vi "Launch Worker.vi"(8 "error in (no error)":errorcluster, 9 "Name":string, 10 "Subordinate Object":refnum<class "Worker.lvclass">, 11 "Application Controller in":refnum<class "Application Controller.lvclass">) -> (0 "error out":errorcluster, 2 "Nested Actor's Enqueuer":refnum<class "Message Enqueuer.lvclass">, 3 "Application Controller out":refnum<class "Application Controller.lvclass">)   [LabVIEW 2016, in "Application Controller.lvclass"]
uses:
  Application Controller.lvclass
  Worker/Worker.lvclass
  C:/github/Measure_core/Template Module/Template Module.lvclass
  <vilib>/ActorFramework/Message Enqueuer/Message Enqueuer.lvclass
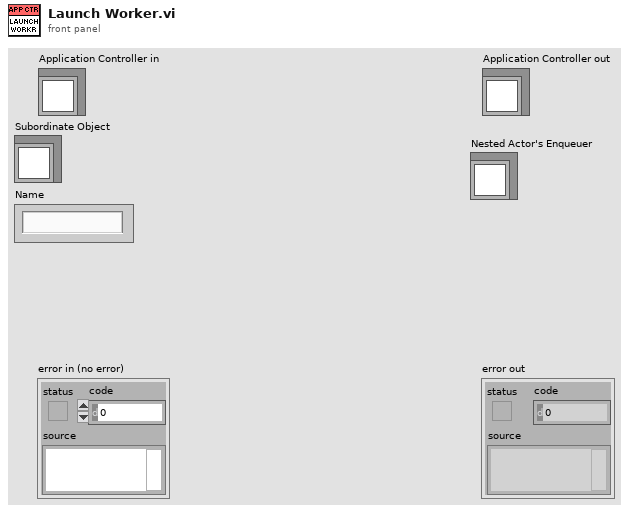
[diagram p1: front panel]
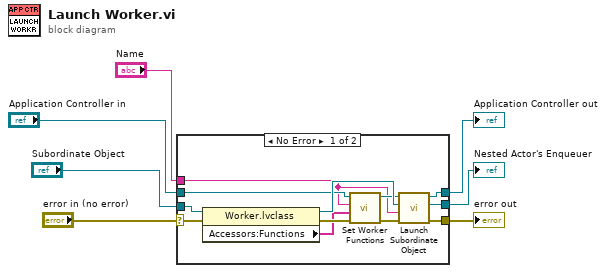
[diagram p0: block diagram]
diagram:
  n1 = case shown="No Error" "error in (no error)" {
    selector: "error in (no error)" -> [w18 w21]
    tunnel: [w17 w21] -> w6
    tunnel: [w19 w20] -> w4
    tunnel: "Application Controller in" -> [w11 w20]
    tunnel: "Subordinate Object" -> [w14 _]
    tunnel: "Name" -> [w9 _]
    tunnel: [w16 _] -> w1
    frame No Error {
      n2 = property class="Worker.lvclass"(reference=w14, error in=w18) -> (reference out=w13:refnum<class "Worker.lvclass">, error out=w15:errorcluster, "Accessors:Functions"=w8:string[])
      n3 = call-dynamic "Set Worker Functions.vi"("error in (no error)"=w15, "Functions"=w8, "Name"=w9, "Application Controller in"=w11) -> ("error out"=w12:errorcluster, "Application Controller out"=w10:refnum<class "Application Controller.lvclass">)  [unwired: 6 in]
      n4 = call-dynamic "Launch Subordinate Object.vi"("error in (no error)"=w12, "Name"=w9, "Subordinate Object"=w13, "Measure Object in"=w10) -> ("error out"=w17:errorcluster, "Nested Actor's Enqueuer"=w16:refnum<class "Message Enqueuer.lvclass">, "Measure Object out"=w19:refnum<class "Application Controller.lvclass">)  [unwired: 5 in]
    }
    frame Error {
    }
  }
  "error out" <- w6
  "Application Controller out" <- w4
  "Nested Actor's Enqueuer" <- w1
